vi "veristandSteps-assemblyProjectFile-update.vi"() -> ()   [LabVIEW 2014, in "veristand-steps-build-system.lvlib"]
uses:
  <vilib>/xml/Load XML File.vi
  <vilib>/xml/Close Reference(Node).vi
  <vilib>/xml/Close Reference(NNMap).vi
  <vilib>/ni/Simple XML/_polymorphics/Create Tag - Child with Text.vi
  veristand-steps-build-system.lvlib
  <vilib>/xml/NI_XML.lvlib
  <resource>/objmgr/DOMUserDefRef.rc
  <vilib>/ni/Simple XML/Simple XML.lvlib
  <vilib>/Wiresmith Technology/LabVIEW CLI/CLI Class/CLI.lvclass
panel:
  out "error out":errorcluster
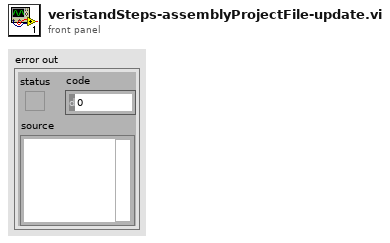
[diagram p1: front panel]
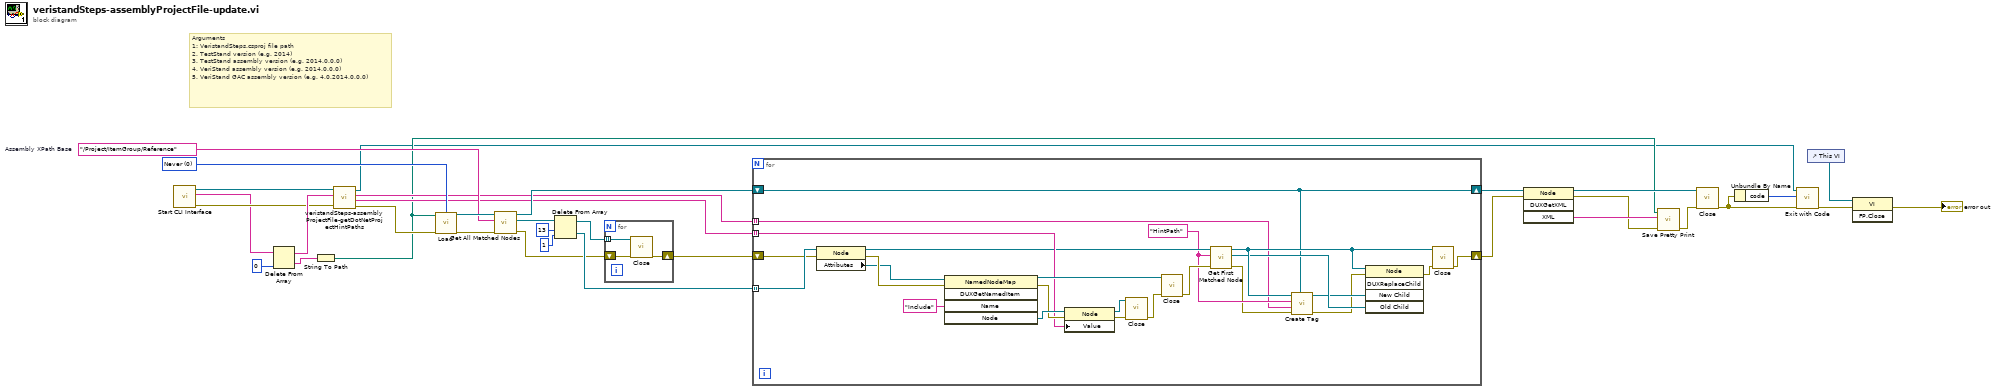
[diagram p0: block diagram]
diagram:
  w31 = "/Project/ItemGroup/Reference"  # Assembly XPath Base
  w34 = 0 items=["Never", "Always", "Auto"] ("validate on load (Auto)")
  # "Arguments\n1: VeristandSteps.csproj file path\n2. TestStand version (e.g. 2014)\n3. TestStand assembly version (e.g. 2014.0.0.0)\n4. VeriStand assembly version (e.g. 2014.0.0.0)\n5. VeriStand GAC assembly version (e.g. 4.0.2014.0.0.0)"
  n1 = call <vilib>:"Start CLI Interface.vi"() -> ("error out"=w10:errorcluster, "Custom Parameters"=w1:string[], "CLI out"=w11:refnum<class "CLI.lvclass">)  [unwired: 9 in]
  n2 = Delete From Array(array=w1, index=0) -> (deleted portion=w13:string, array with subset deleted=w12:string[])  [unwired: 1 in]
  n3 = String To Path(string=w13) -> (path=w6:path)
  n4 = call "veristandSteps-assemblyProjectFile-getDotNetProjectHintPaths.vi"("error in"=w10, "Parameters"=w12, "CLI in"=w11) -> ("error out"=w9:errorcluster, "New Assembly Include Paths"=w8:string[], "New Assembly Hint Paths"=w7:string[], "CLI out"=w2:refnum<class "CLI.lvclass">)  [unwired: 5 in]
  n5 = call-poly <vilib>:"Load.vi"("path to XML document"=w6, "validate on load (Auto)"=w34, "error in (no error)"=w9) -> ("DOM document out"=w32:refnum<k20>, "error out"=w33:errorcluster)  [unwired: 10 in, 1 out]
  n6 = call <vilib>:"Get All Matched Nodes.vi"("error in (no error)"=w33, "XPath expression"=w31, "node in"=w32) -> ("error out"=w25:errorcluster, "node result array"=w30:refnum<k20>[], "node out"=w18:refnum<k20>)  [unwired: 6 in]
  n7 = Delete From Array(array=w30, length=13, index=1 ("length")) -> (deleted portion=w27:refnum<k20>[], array with subset deleted=w26:refnum<k20>[])
  n8 = for {
    tunnel: w26 -> [w37] mode=indexing
    shift-right: [w35] -> w24
    shift-left: w25 -> [w36]
    n9 = call-poly <vilib>:"Close.vi"("error in (no error)"=w36, "node"=w37) -> ("error out"=w35:errorcluster)  [unwired: 7 in]
  }
  n10 = for {
    tunnel: w27 -> [w58] mode=indexing
    shift-right: [w52] -> w23
    shift-left: w24 -> [w57]
    tunnel: w8 -> [w51] mode=indexing
    tunnel: w7 -> [w39] mode=indexing
    shift-right: [w38] -> w17
    shift-left: w18 -> [w38]
    w46 = "HintPath" ("XPath expression")
    n11 = property class="Node"(reference=w58, error in=w57) -> (reference out=w47:refnum<k20>, error out=w61:errorcluster, "Attributes"=w59:refnum<k20>)
    n12 = invoke class="NamedNodeMap" method="DUXGetNamedItem"(reference=w59, error in=w61, "Name"="Include") -> (reference out=w53:refnum<k20>, error out=w55:errorcluster, "Node"=w56:refnum<k20>)  [unwired: 2 in, 2 out]
    n13 = property class="Node"(reference=w56, error in=w55, "Value"=w51) -> (reference out=w54:refnum<k20>, error out=w50:errorcluster)
    n14 = call-poly <vilib>:"Close.vi"("error in (no error)"=w50, "node"=w54) -> ("error out"=w49:errorcluster)  [unwired: 7 in]
    n15 = call-poly <vilib>:"Close.vi"("error in (no error)"=w49, "named node map"=w53) -> ("error out"=w48:errorcluster)  [unwired: 7 in]
    n16 = call <vilib>:"Get First Matched Node.vi"("error in (no error)"=w48, "XPath expression"=w46, "node in"=w47) -> ("error out"=w45:errorcluster, "node result"=w43:refnum<k20>, "node out"=w44:refnum<k20>)  [unwired: 6 in]
    n17 = call-poly <vilib>:"Create Tag.vi"("DOM document reference"=w38, "error in (no error)"=w45, "Text Data"=w39, "Tag Name"=w46, "Parent Element reference"=w44) -> ("error out"=w41:errorcluster, "Child Element reference"=w42:refnum<k20>)  [unwired: 5 in]
    n18 = invoke class="Node" method="DUXReplaceChild"(reference=w44, error in=w41, "New Child"=w42, "Old Child"=w43) -> (error out=w40:errorcluster)  [unwired: 1 in, 4 out]
    n19 = call-poly <vilib>:"Close.vi"("error in (no error)"=w40, "node"=w44) -> ("error out"=w52:errorcluster)  [unwired: 7 in]
  }
  n20 = invoke class="Node" method="DUXGetXML"(reference=w17, error in=w23) -> (reference out=w19:refnum<k20>, error out=w21:errorcluster, "XML"=w22:string)  [unwired: 2 in, 1 out]
  n21 = call <vilib>:"Save Pretty Print.vi"("error in (no error)"=w21, "Pretty XML String"=w22, "XML file path"=w6) -> ("error out"=w20:errorcluster)  [unwired: 7 in, 1 out]
  n22 = call-poly <vilib>:"Close.vi"("error in (no error)"=w20, "node"=w19) -> ("error out"=w4:errorcluster)  [unwired: 7 in]
  n23 = Unbundle By Name(w4) -> ("code"=w3:i32)
  n24 = call <vilib>:"Exit with Code.vi"("error in (no error)"=w4, "Exit Code (0)"=w3, "CLI in"=w2) -> ("error out"=w5:errorcluster)  [unwired: 8 in]
  n25 = control-ref of="This VI"() -> (w15:refnum<vi>)
  n26 = invoke class="VI" method="FP.Close"(reference=w15, error in=w5) -> (error out=→"error out":errorcluster)  [unwired: 1 in, 2 out]
